vi "ge_FilterMeasSpeed.vi"(8 "error in":errorcluster, 10 "MeasType":T1=enum."Dynamic", 11 "Rate Class":refnum<vi>) -> (0 "error out":errorcluster)   [LabVIEW 2012]
uses:
  Custom Ctrls/ge_MeasType.ctl
  Common/Controls/TE_Designator.ctl
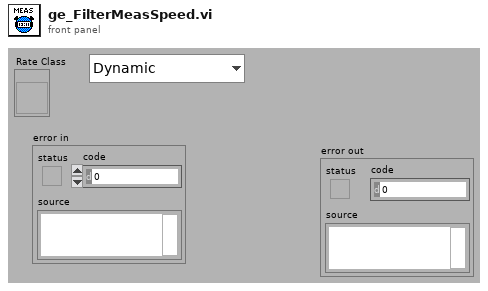
[diagram p1: front panel]
types:
  T1 = typedef "ge_MeasType.ctl" = enum16{"Voltage", "Frequency", "Tachometer", "Dynamic", "Thermocouple", "RTD", "Strain", "Current", "Resistance"}
  T2 = enum8{"Enabled", "Disabled", "Disabled and Grayed Out"}
  T3 = typedef "TE_Designator.ctl" = enum16{"High Speed", "Low Speed"}
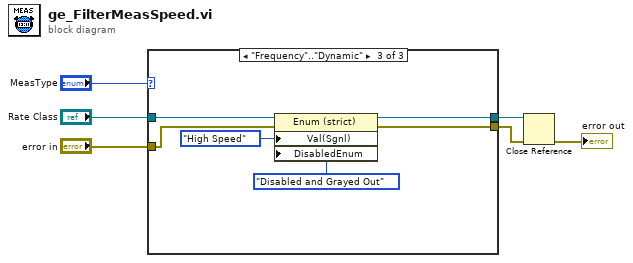
[diagram p0: block diagram]
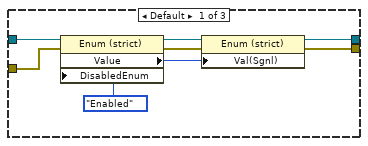
[diagram p2: hidden frame]
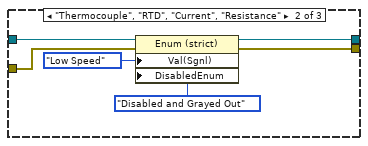
[diagram p3: hidden frame]
diagram:
  n1 = case shown="\"Frequency\"..\"Dynamic\"" "MeasType" {
    tunnel: "Rate Class" -> [w14 w20 w26]
    tunnel: [w9 w16 w23] -> w4
    tunnel: [w8 w15 w22] -> w3
    tunnel: "error in" -> [w7 w17 w21]
    frame Default {
      n2 = property class="Enum (strict)"(reference=w14, error in=w7, "DisabledEnum"=T2."Enabled" ("Disabled")) -> (reference out=w12:refnum<vi>, error out=w11:errorcluster, "Value"=w10:enum16{"High Speed", "Low Speed"})
      n3 = property class="Enum (strict)"(reference=w12, error in=w11, "Val(Sgnl)"=w10) -> (reference out=w9:refnum<vi>, error out=w8:errorcluster)
    }
    frame "Thermocouple", "RTD", "Current", "Resistance" {
      n4 = property class="Enum (strict)"(reference=w20, error in=w17, "Val(Sgnl)"=TE_Designator."Low Speed" ("Value"), "DisabledEnum"=T2."Disabled and Grayed Out" ("Disabled")) -> (reference out=w16:refnum<vi>, error out=w15:errorcluster)
    }
    frame "Frequency".."Dynamic" {
      n5 = property class="Enum (strict)"(reference=w26, error in=w21, "Val(Sgnl)"=TE_Designator."High Speed" ("Value"), "DisabledEnum"=T2."Disabled and Grayed Out" ("Disabled")) -> (reference out=w23:refnum<vi>, error out=w22:errorcluster)
    }
  }
  n6 = Close Reference(reference=w4, error in (no error)=w3) -> (error out=→"error out":errorcluster)
